vi "Start Stop.vi"(8 "error in (no error)":errorcluster, 10 "Start/stop":bool, 11 "GUI_Graph in":refnum<class "GUI_Graph.lvclass">) -> (0 "error out":errorcluster, 3 "GUI_Graph out":refnum<class "GUI_Graph.lvclass">)   [LabVIEW 2020, in "GUI_Graph.lvlib" / "GUI_Graph.lvclass"]
uses:
  GUI_Graph.lvclass
  GUI_Graph.lvclass/GUI_Graph.ctl
  Measurement/Measurement Messages/START STOP Msg/START STOP Msg.lvclass/START STOP Msg.ctl
  <vilib>/ActorFramework/Message Enqueuer/Message Enqueuer.lvclass/Message Enqueuer.ctl
  <vilib>/ActorFramework/Message Enqueuer/Enqueue.vi
  Measurement/Measurement Messages/START STOP Msg/START STOP Msg.lvclass
  C:/Program Files/National Instruments/LabVIEW 2020/vi.lib/ActorFramework/Message/Message.lvclass
  <vilib>/ActorFramework/Message Priority Queue/Priority Enqueue.vi
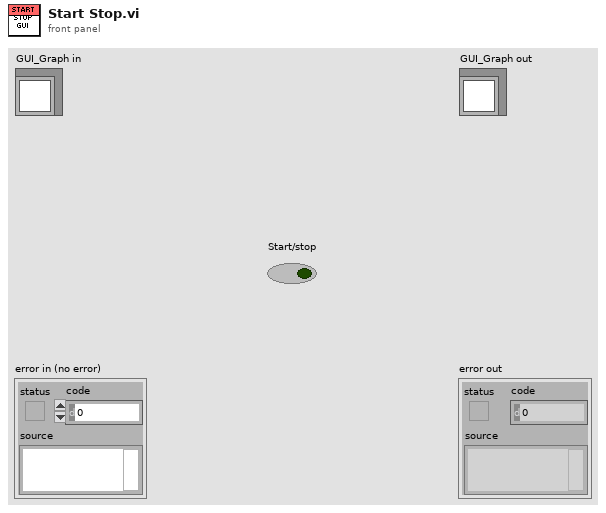
[diagram p1: front panel]
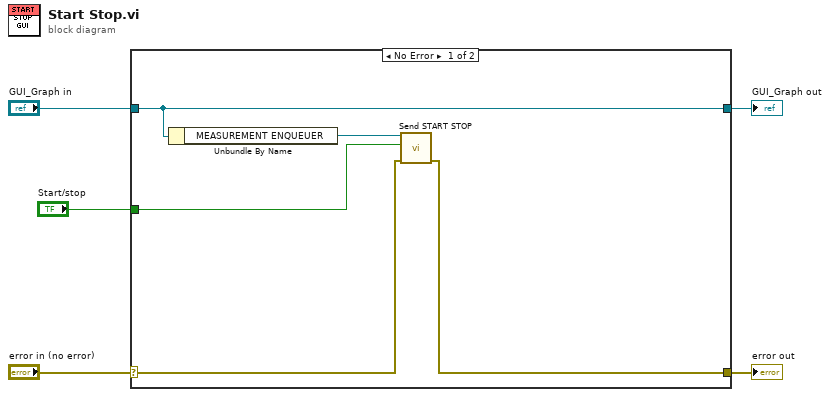
[diagram p0: block diagram]
diagram:
  n1 = case shown="No Error" "error in (no error)" {
    selector: "error in (no error)" -> [w7 w12]
    tunnel: [w6 w12] -> w4
    tunnel: [w10 w11] -> w2
    tunnel: "GUI_Graph in" -> [w10 w11]
    tunnel: "Start/stop" -> [w8 _]
    frame No Error {
      n2 = Unbundle By Name(w10) -> ("MEASUREMENT ENQUEUER"=w9:refnum<class "Message Enqueuer.lvclass">)
      n3 = call "Send START STOP.vi"("error in (no error)"=w7, "Start/stop"=w8, "Message Enqueuer"=w9) -> ("error out"=w6:errorcluster)  [unwired: 7 in, 1 out]
    }
    frame Error {
    }
  }
  "error out" <- w4
  "GUI_Graph out" <- w2
